vi "Calculator.vi"() -> ()   [LabVIEW 2020]
panel:
  in  "stop":bool
  out "A / B":dbl
  out "A x B":dbl
  out "A - B":dbl
  out "A + B":dbl
  in  "B":dbl
  in  "A":dbl
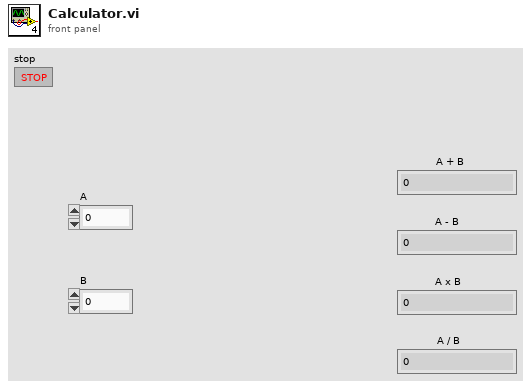
[diagram p1: front panel]
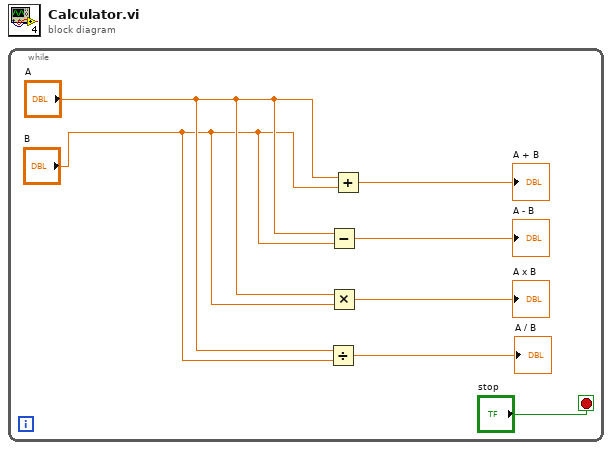
[diagram p0: block diagram]
diagram:
  n1 = while {
    stop <- "stop" stop-if-true
    n2 = Divide(x="A", y="B") -> (x/y=→"A / B":dbl)
    n3 = Subtract(x="A", y="B") -> (x-y=→"A - B":dbl)
    n4 = Multiply(x="A", y="B") -> (x*y=→"A x B":dbl)
    n5 = Add(x="A", y="B") -> (x+y=→"A + B":dbl)
  }
